vi "BuildDescription.vi"(2 "MyState":T1, 3 "ROS in":T2={"topic port"=1236, "Node"="/labview", "topic"="/robot/head/command_head_nod", "type"="std_msgs/Bool", "node port"=7000, "error "={"status"=FALSE, "code"=0, "source"=""}, "Direction"=enum."Publisher", "APIs"=[], "Update (ms)"=1, "write queue"=1}) -> (1 "Setup":string)   [LabVIEW 2012]
uses:
  SubVIs/_ROSDirection.ctl
  SubVIs/_ROSControl.ctl
  MyState.ctl
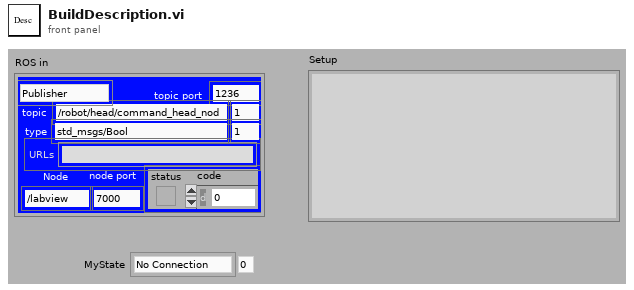
[diagram p1: front panel]
types:
  T1 = typedef "MyState.ctl" = enum16{"No Connection", "Registered", "Connected", "Close"}
  T2 = typedef "_ROSControl.ctl" = cluster{"topic port":u16, "Node":string, "topic":string, "type":string, "node port":u32, "error ":errorcluster, "Direction":T3, "APIs":string[], "Update (ms)":u16, "write queue":u16}
  T3 = typedef "_ROSDirection.ctl" = enum16{"Node", "Publisher", "Subscriber", "Service Client"}
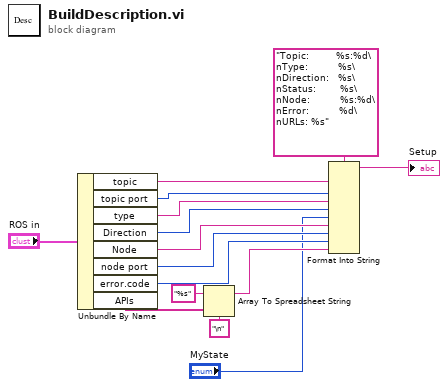
[diagram p0: block diagram]
diagram:
  n1 = Unbundle By Name("ROS in") -> ("topic"=w14:string, "topic port"=w13:u16, "type"=w12:string, "Direction"=w11:T3, "Node"=w3:string, "node port"=w10:u32, "error.code"=w9:i32, "APIs"=w7:string[])
  n2 = Array To Spreadsheet String(delimiter (Tab)="\n", array=w7, 3:"%s" ("format string")) -> (spreadsheet string=w8:string)
  n3 = Format Into String(format string="Topic:         %s:%d\nType:          %s\nDirection:   %s\nStatus:        %s\nNode:          %s:%d\nError:          %d\nURLs: %s", w14, w13, w12, w11, "MyState", w3, w10, w9, w8) -> (resulting string=→"Setup":string)  [unwired: 2 in, 1 out]
